vi "WaitOnTestComplete.vi"(8 "error in (no error)":errorcluster, 11 "TestCase in":refnum<class "TestCase.lvclass">) -> (0 "error out":errorcluster, 3 "TestCase out":refnum<class "TestCase.lvclass">)   [LabVIEW 2011, in "TestCase.lvclass"]
doc: "Insert WaitOnTestComplete at the end of setUp test hook if the test hook VI opens any references that are needed by the test methods at run time."
uses:
  TestCase.lvclass
  TestCase.lvclass/TestCase.ctl
panel:
  # "JKI VI Tester for LabVIEW\nhttp://jkisoft.com/vi-tester\nCopyright (C) 2007-2009, JKI <info@jkisoft.com>\nALL RIGHTS RESERVED"
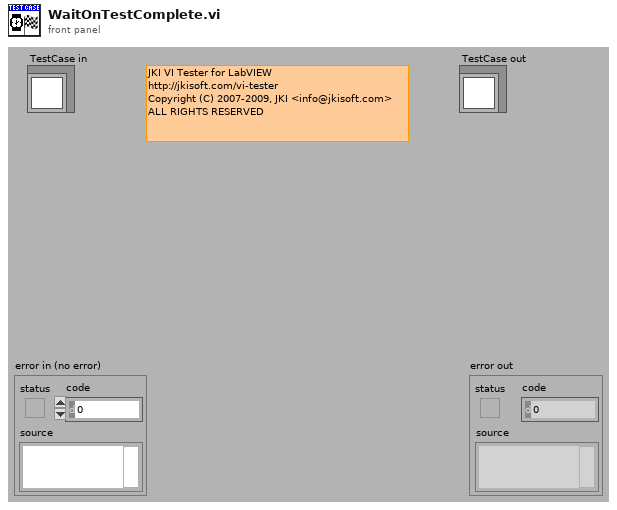
[diagram p1: front panel]
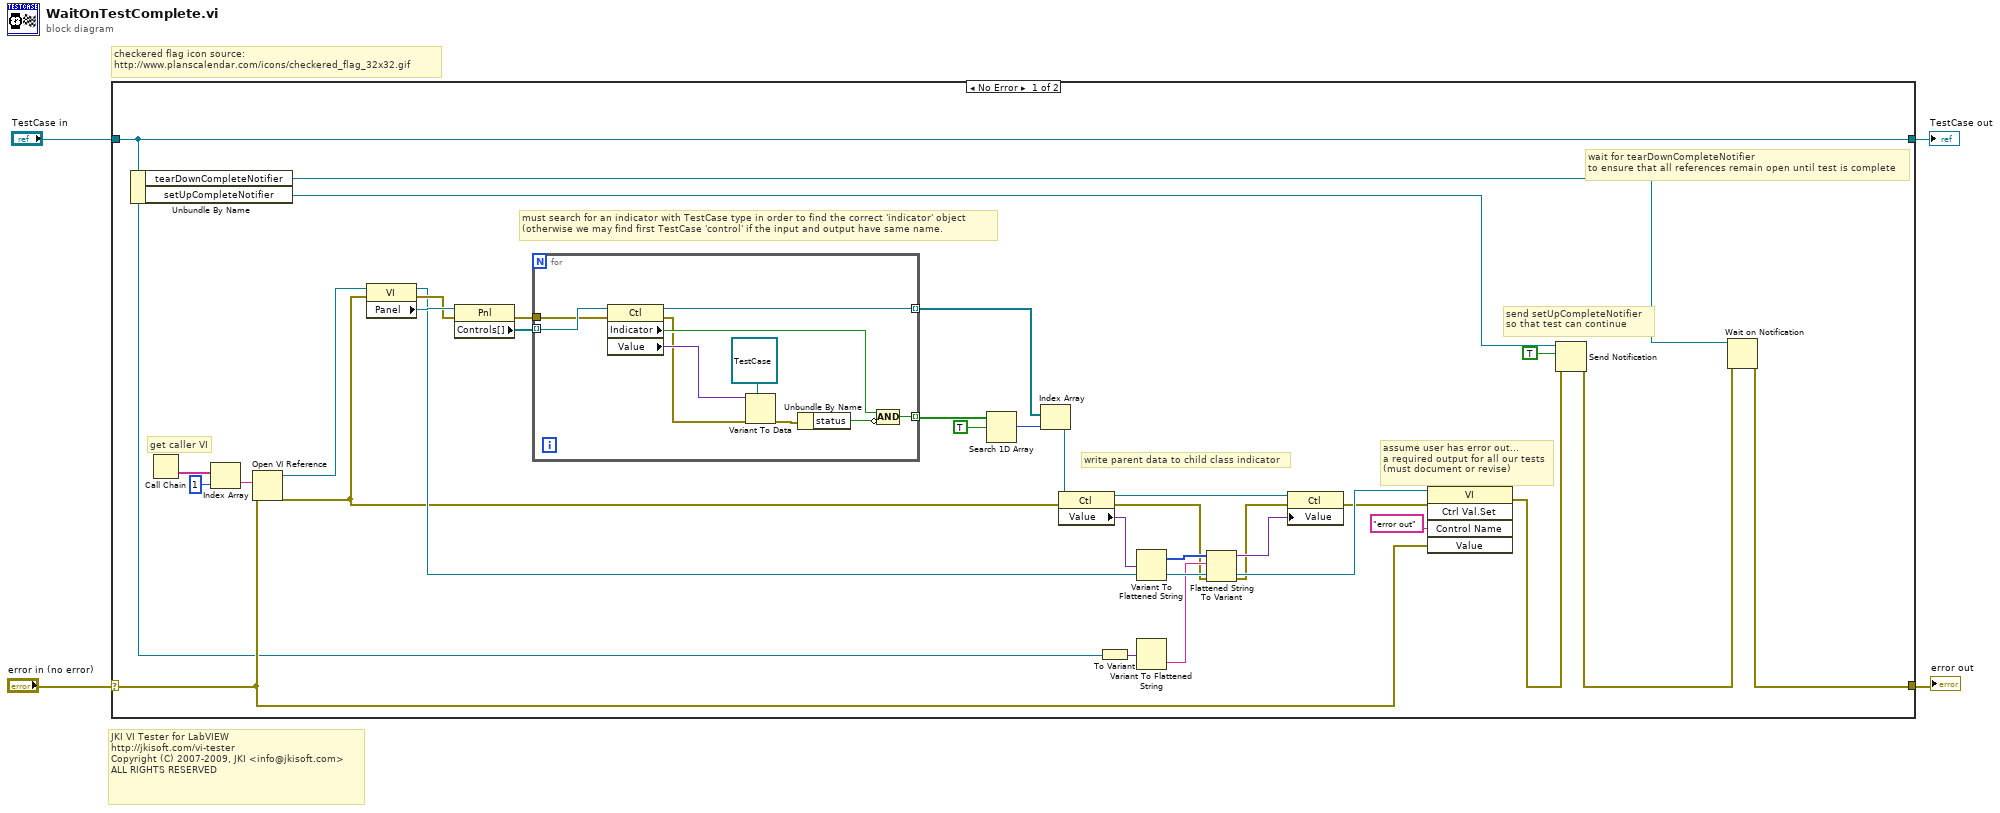
[diagram p0: block diagram]
diagram:
  # "JKI VI Tester for LabVIEW\nhttp://jkisoft.com/vi-tester\nCopyright (C) 2007-2009, JKI <info@jkisoft.com>\nALL RIGHTS RESERVED"
  # "checkered flag icon source:\nhttp://www.planscalendar.com/icons/checkered_flag_32x32.gif"
  n1 = case shown="No Error" "error in (no error)" {
    selector: "error in (no error)" -> [w18 w49]
    tunnel: [w36 w49] -> w3
    tunnel: [w7 w48] -> w1
    tunnel: "TestCase in" -> [w7 w48]
    frame No Error {
      # "write parent data to child class indicator"
      # "get caller VI"
      # "must search for an indicator with TestCase type in order to find the correct 'indicator' object\n(otherwise we may find first TestCase 'control' if the input and output have same name."
      # "assume user has error out...\na required output for all our tests\n(must document or revise)"
      # "wait for tearDownCompleteNotifier\nto ensure that all references remain open until test is complete"
      # "send setUpCompleteNotifier\nso that test can continue"
      n2 = Unbundle By Name(w7) -> ("tearDownCompleteNotifier"=w37:refnum<notifier>, "setUpCompleteNotifier"=w35:refnum<notifier>)
      n3 = Call Chain() -> (call chain=w32:string[])
      n4 = Index Array(array=w32, index=1) -> (element=w30:string)
      n5 = Open VI Reference(vi path=w30, error in (no error)=w18) -> (vi reference=w17:refnum<vi>, error out=w8:errorcluster)  [unwired: 4 in]
      n6 = property class="VI"(reference=w17, error in=w8) -> (reference out=w20:refnum<vi>, error out=w27:errorcluster, "Panel"=w29:refnum<vi>)
      n7 = property class="Pnl"(reference=w29, error in=w27) -> (error out=w26:errorcluster, "Controls[]"=w28:refnum<vi>[])  [unwired: 1 out]
      n8 = for {
        tunnel: w28 -> [w47] mode=indexing
        tunnel: [w41] -> w25 mode=indexing
        tunnel: w26 -> [w39]
        tunnel: [w38] -> w22 mode=indexing
        n9 = property class="Ctl"(reference=w47, error in=w39) -> (reference out=w38:refnum<vi>, error out=w40:errorcluster, "Indicator"=w42:bool, "Value"=w45:variant)
        n10 = Variant To Data(error in=w40, type=refnum<class "TestCase.lvclass"> refnum ("TestCase.lvclass"), Variant=w45) -> (error out=w44:errorcluster)  [unwired: 1 out]
        n11 = Unbundle By Name(w44) -> ("status"=w43:bool)
        n12 = Compound Arithmetic op=AND(w42, invert w43) -> (w41:bool)
      }
      n13 = Search 1D Array(1D array=w25, element=TRUE) -> (index of element=w23:i32)  [unwired: 1 in]
      n14 = Index Array(array=w22, index=w23) -> (element=w5:refnum<vi>)
      n15 = property class="Ctl"(reference=w5, error in=w8) -> (reference out=w13:refnum<vi>, error out=w10:errorcluster, "Value"=w16:variant)
      n16 = To Variant(anything=w7) -> (Variant=w11:variant)
      n17 = Variant To Flattened String(Variant=w16) -> (1:w15:i16[])  [unwired: 1 out]
      n18 = Variant To Flattened String(Variant=w11) -> (data string=w14:string)  [unwired: 1 out]
      n19 = Flattened String To Variant(4:w10, 6:w14, 7:w15) -> (0:w9:errorcluster, 3:w12:variant)
      n20 = property class="Ctl"(reference=w13, error in=w9, "Value"=w12) -> (error out=w6:errorcluster)  [unwired: 1 out]
      n21 = invoke class="VI" method="Ctrl Val.Set"(reference=w20, error in=w6, "Control Name"="error out", "Value"=w18) -> (error out=w19:errorcluster)  [unwired: 1 in, 4 out]
      n22 = Send Notification(notification=TRUE, notifier=w35, error in (no error)=w19) -> (error out=w34:errorcluster)  [unwired: 1 out]
      n23 = Wait on Notification(notifier=w37, error in (no error)=w34) -> (error out=w36:errorcluster)  [unwired: 2 in, 3 out]
    }
    frame Error {
    }
  }
  "error out" <- w3
  "TestCase out" <- w1
